vi "export_DFX.vi"(0 "vacuum":sgl, 1 "Q1":sgl, 2 "P@Q1":sgl, 3 "Q2":sgl, 4 "P@Q2":sgl, 5 "Pmxax":sgl, 6 "dfx file name":string, 7 "Ploose":bool) -> ()   [LabVIEW 2014]
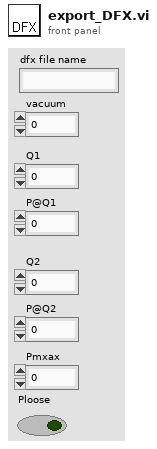
[diagram p1: front panel]
types:
  T1 = enum16{"open", "replace", "create", "open or create", "replace or create", "replace or create with confirmation"}
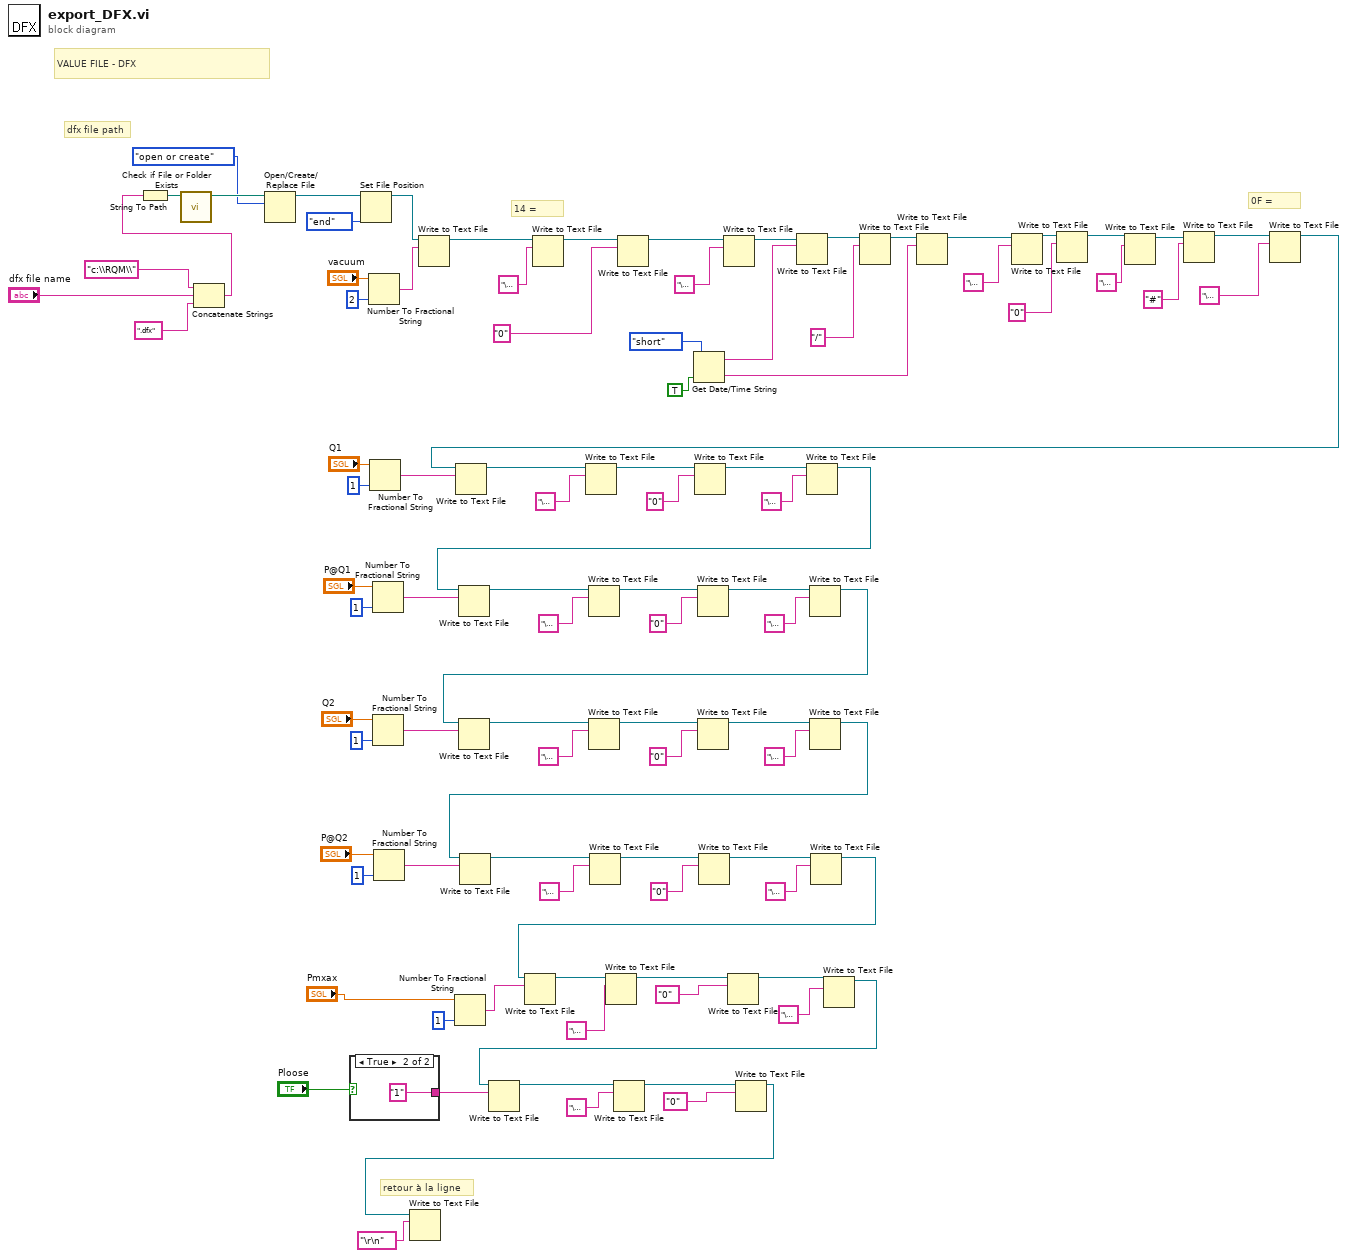
[diagram p0: block diagram]
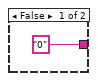
[diagram p2: hidden frame]
diagram:
  # "0F ="
  # "14 ="
  # "dfx file path"
  # "VALUE FILE - DFX"
  # "retour à la ligne"
  n1 = Concatenate Strings("c:\\RQM\\", "dfx file name", ".dfx") -> (w44:string)
  n2 = String To Path(string=w44) -> (path=w96:path)
  n3 = call <vilib>:"Check if File or Folder Exists.vi"("path"=w96) -> ("dup path"=w74:path)  [unwired: 8 in, 2 out]
  n4 = Open/Create/Replace File(file path (use dialog)=w74, operation (0:open)=T1."open or create") -> (refnum out=w72:refnum<file>)  [unwired: 4 in, 2 out]
  n5 = case shown="True" "Ploose" {
    tunnel: ["0" "1"] -> w9
    frame False {
    }
    frame True {
    }
  }
  n6 = Set File Position(refnum=w72, from (0:start)=enum16{"start", "end", "current"}."end") -> (refnum out=w71:refnum<file>)  [unwired: 2 in, 1 out]
  n7 = Number To Fractional String(number="vacuum", precision (6)=i16 2 ("width (-)")) -> (F-format string=w75:string)  [unwired: 2 in]
  n8 = Number To Fractional String(number="Q1", precision (6)=i16 1 ("width (-)")) -> (F-format string=w64:string)  [unwired: 2 in]
  n9 = Number To Fractional String(number="P@Q1", precision (6)=i16 1 ("width (-)")) -> (F-format string=w42:string)  [unwired: 2 in]
  n10 = Number To Fractional String(number="Q2", precision (6)=i16 1 ("width (-)")) -> (F-format string=w32:string)  [unwired: 2 in]
  n11 = Number To Fractional String(number="P@Q2", precision (6)=i16 1 ("width (-)")) -> (F-format string=w22:string)  [unwired: 2 in]
  n12 = Write to Text File(file (use dialog)=w71, text=w75) -> (refnum out=w95:refnum<file>)  [unwired: 2 in, 2 out]
  n13 = Number To Fractional String(number="Pmxax", precision (6)=i16 1 ("width (-)")) -> (F-format string=w54:string)  [unwired: 2 in]
  n14 = Write to Text File(file (use dialog)=w95, text="\u0014") -> (refnum out=w92:refnum<file>)  [unwired: 2 in, 2 out]
  n15 = Write to Text File(file (use dialog)=w92, text="0") -> (refnum out=w91:refnum<file>)  [unwired: 2 in, 2 out]
  n16 = Get Date/Time String(date format (0)=enum16{"short", "long", "abbreviated"}."short", want seconds? (F)=TRUE) -> (date string=w87:string, time string=w86:string)  [unwired: 1 in]
  n17 = Write to Text File(file (use dialog)=w91, text="\u0014") -> (refnum out=w88:refnum<file>)  [unwired: 2 in, 2 out]
  n18 = Write to Text File(file (use dialog)=w88, text=w87) -> (refnum out=w83:refnum<file>)  [unwired: 2 in, 2 out]
  n19 = Write to Text File(file (use dialog)=w83, text="/") -> (refnum out=w82:refnum<file>)  [unwired: 2 in, 2 out]
  n20 = Write to Text File(file (use dialog)=w82, text=w86) -> (refnum out=w85:refnum<file>)  [unwired: 2 in, 2 out]
  n21 = Write to Text File(file (use dialog)=w85, text="\u0014") -> (refnum out=w79:refnum<file>)  [unwired: 2 in, 2 out]
  n22 = Write to Text File(file (use dialog)=w79, text="0") -> (refnum out=w66:refnum<file>)  [unwired: 2 in, 2 out]
  n23 = Write to Text File(file (use dialog)=w66, text="\u0014") -> (refnum out=w65:refnum<file>)  [unwired: 2 in, 2 out]
  n24 = Write to Text File(file (use dialog)=w65, text="#" ("string")) -> (refnum out=w78:refnum<file>)  [unwired: 2 in, 2 out]
  n25 = Write to Text File(file (use dialog)=w78, text="\u000f") -> (refnum out=w55:refnum<file>)  [unwired: 2 in, 2 out]
  n26 = Write to Text File(file (use dialog)=w55, text=w64) -> (refnum out=w58:refnum<file>)  [unwired: 2 in, 2 out]
  n27 = Write to Text File(file (use dialog)=w58, text="\u0014") -> (refnum out=w59:refnum<file>)  [unwired: 2 in, 2 out]
  n28 = Write to Text File(file (use dialog)=w59, text="0") -> (refnum out=w56:refnum<file>)  [unwired: 2 in, 2 out]
  n29 = Write to Text File(file (use dialog)=w56, text="\u000f") -> (refnum out=w33:refnum<file>)  [unwired: 2 in, 2 out]
  n30 = Write to Text File(file (use dialog)=w33, text=w42) -> (refnum out=w37:refnum<file>)  [unwired: 2 in, 2 out]
  n31 = Write to Text File(file (use dialog)=w37, text="\u0014") -> (refnum out=w38:refnum<file>)  [unwired: 2 in, 2 out]
  n32 = Write to Text File(file (use dialog)=w38, text="0") -> (refnum out=w35:refnum<file>)  [unwired: 2 in, 2 out]
  n33 = Write to Text File(file (use dialog)=w35, text="\u000f") -> (refnum out=w23:refnum<file>)  [unwired: 2 in, 2 out]
  n34 = Write to Text File(file (use dialog)=w23, text=w32) -> (refnum out=w27:refnum<file>)  [unwired: 2 in, 2 out]
  n35 = Write to Text File(file (use dialog)=w27, text="\u0014") -> (refnum out=w28:refnum<file>)  [unwired: 2 in, 2 out]
  n36 = Write to Text File(file (use dialog)=w28, text="0") -> (refnum out=w25:refnum<file>)  [unwired: 2 in, 2 out]
  n37 = Write to Text File(file (use dialog)=w25, text="\u000f") -> (refnum out=w13:refnum<file>)  [unwired: 2 in, 2 out]
  n38 = Write to Text File(file (use dialog)=w13, text=w22) -> (refnum out=w17:refnum<file>)  [unwired: 2 in, 2 out]
  n39 = Write to Text File(file (use dialog)=w17, text="\u0014") -> (refnum out=w18:refnum<file>)  [unwired: 2 in, 2 out]
  n40 = Write to Text File(file (use dialog)=w18, text="0") -> (refnum out=w15:refnum<file>)  [unwired: 2 in, 2 out]
  n41 = Write to Text File(file (use dialog)=w15, text="\u000f") -> (refnum out=w12:refnum<file>)  [unwired: 2 in, 2 out]
  n42 = Write to Text File(file (use dialog)=w12, text=w54) -> (refnum out=w50:refnum<file>)  [unwired: 2 in, 2 out]
  n43 = Write to Text File(file (use dialog)=w50, text="\u0014") -> (refnum out=w49:refnum<file>)  [unwired: 2 in, 2 out]
  n44 = Write to Text File(file (use dialog)=w49, text="0") -> (refnum out=w8:refnum<file>)  [unwired: 2 in, 2 out]
  n45 = Write to Text File(file (use dialog)=w8, text="\u000f") -> (refnum out=w7:refnum<file>)  [unwired: 2 in, 2 out]
  n46 = Write to Text File(file (use dialog)=w7, text=w9) -> (refnum out=w3:refnum<file>)  [unwired: 2 in, 2 out]
  n47 = Write to Text File(file (use dialog)=w3, text="\u0014") -> (refnum out=w4:refnum<file>)  [unwired: 2 in, 2 out]
  n48 = Write to Text File(file (use dialog)=w4, text="0") -> (refnum out=w2:refnum<file>)  [unwired: 2 in, 2 out]
  n49 = Write to Text File(file (use dialog)=w2, text="\r\n") -> ()  [unwired: 2 in, 3 out]
